vi "RMAD config.vi"() -> ()   [LabVIEW 2017]
panel:
  in  "Tab Control":T1(tab)
  out "Mote Status":T2(array[cluster]) {"mote state" items=["Lost"=0, "Negotiating"=1, "Operational"=4]}
  out "Link status":T3(array[cluster])
  in  "Send Reset":bool
  in  "SetAUX":bool
  in  "Node":u8=1
  in  "Get Status":bool
  in  "AUX min int":u16=15
  out "AUX data":T4(array[cluster]) {"Node configuration"."configuration" items=[""=100, "Repeater"=0, "Geofon"=1, "Sensor"=2, "Jernbane"=3, "Infralyd"=4]; "Node configuration"."radio config" items=[""=100, "Smartmesh IP"=0]; "batt(V)" format="%.3g"; "temp(c)" format="%.1g"; "?" format="%#.5g"}
  out "Is Logging":T5(array[cluster])
  in  "Adjustable Parameters":T6(array[cluster]) {"ACMP0 ch" items=["Geo 1"=0, "Geo 2"=3]; "ACMP1 ch" items=["Geo 3"=2, "Geo 4"=3]}
  in  "Get Adjustable Params":bool
  in  "Set adjust parameters":bool
  in  "Node":i32=1
  out "NGI Packets Dust":cluster{"MAc Adress":string, "data":string}[](array[cluster])
  out "dust manager mac adress":string
  out "mac adress":string[](array[string])
  out "radio IO":errorcluster
  in  "stop":bool
  out "iteration":i32
  out "gateway IP":T7={"serial_mux IP"="127.0.0.1", "serial_mux port"=9900}
  out "sec since last packet":dbl
  out "node names":string[](array[string])
  in  "initfile":string="rmad config svv.ini"
  in  "stress testing enabled":bool
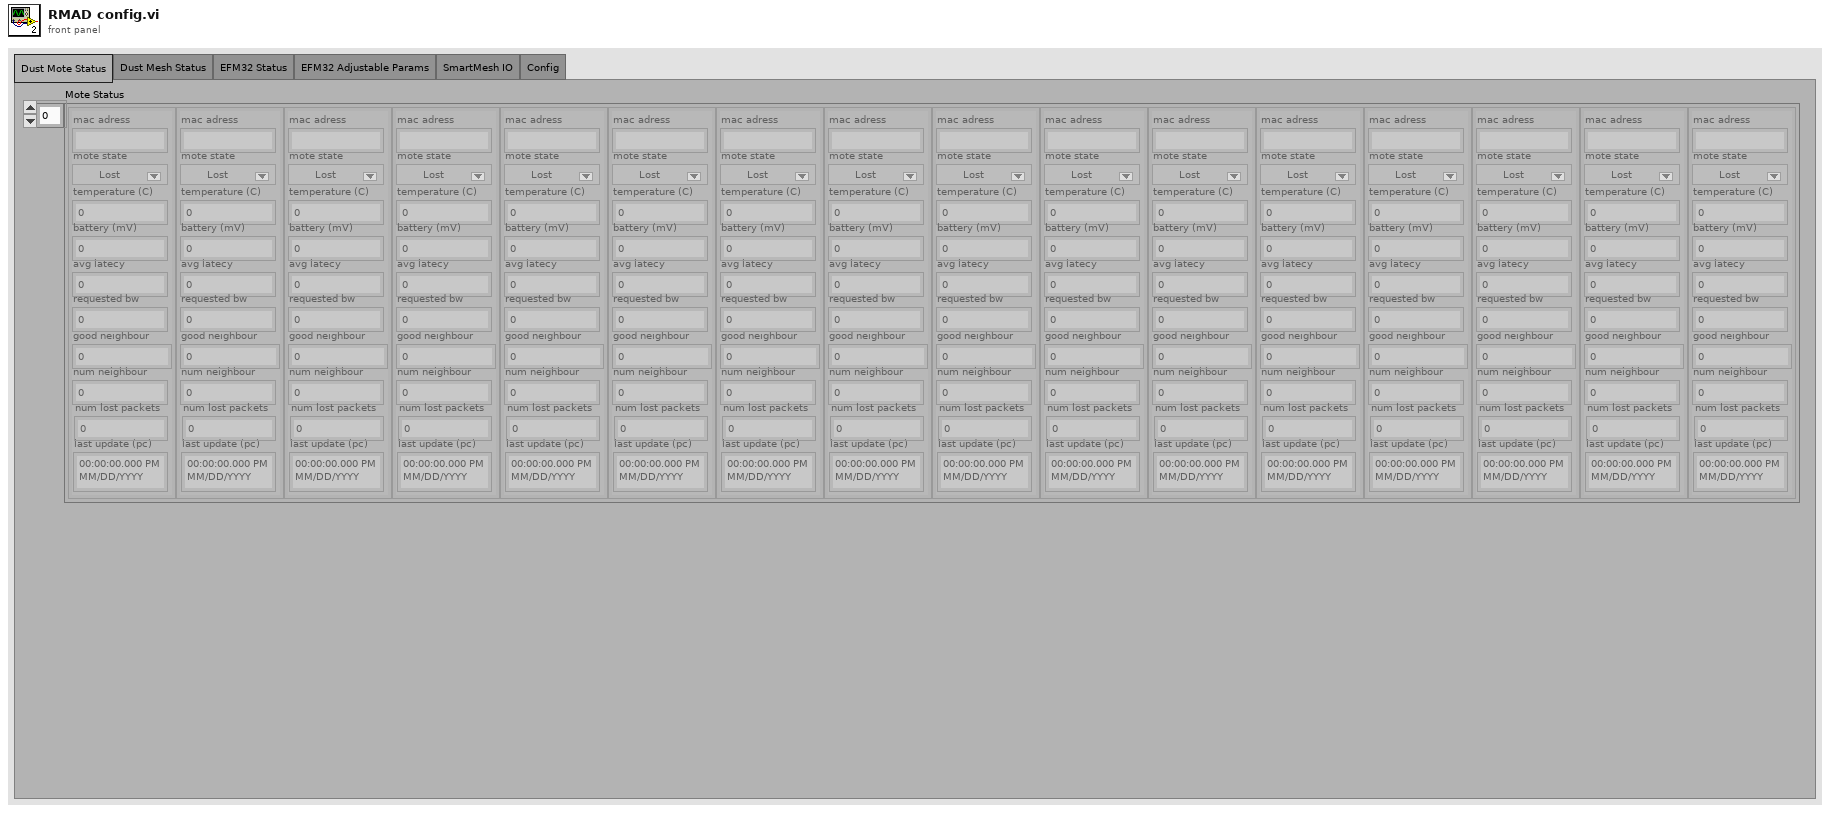
[diagram p1: front panel]
types:
  T1 = enum32{"Dust Mote Status", "Dust Mesh Status", "EFM32 Status", "EFM32 Adjustable Params", "SmartMesh IO", "Config"}
  T2 = cluster{"mac adress":string, "mote state":u8, "temperature (C)":i8, "battery (mV)":u16, "avg latecy":u32, "requested bw":u32, "good neighbour":u8, "num neighbour":u8, "num lost packets":u8, "last update (pc)":timestamp}[]
  T3 = cluster{"source mac adress":string, cluster{"destination":string, "rssi":i8, "TxPackets":u16}[], "last update":timestamp}[]
  T4 = cluster{"Node configuration":cluster{"configuration":u8, "sw ver":u8, "hw rev":u8, "radio config":u8}, "flaggs":bool[], "batt(V)":dbl, "temp(c)":dbl, "is singed int?":bool[], dbl[], "last update (pc)":timestamp}[]
  T5 = cluster{"Is logging":bool, "num avalanch":u16, "logging startet":timestamp}[]
  T6 = cluster{"Min samples":u32, "Samp after cont":u32, "Max samples":u32, "A1 std lim":sgl, "A2 std lim":sgl, "A3 std lim":sgl, "A4 std lim":sgl, "A1 cont lim":sgl, "A2 cont lim":sgl, "A3 cont lim":sgl, "A4 cont lim":sgl, "trigg level":u32, "sample delay":u32, "ACMP0 ch":u8, "ACMP1 ch":u8, "amp trigg":u16, "amp logging":u16}[]
  T7 = cluster{"serial_mux IP":string, "serial_mux port":u16}
  T8 = enum16{"big-endian, network order", "native, host order", "little-endian"}
  T9 = typedef "LVDateTimeRec.ctl" = cluster{"fractional second":dbl, "second":i32, "minute":i32, "hour":i32, "day of month":i32, "month":i32, "year":i32, "day of week":i32, "day of year":i32, "DST":i32}
  T10 = cluster{"Device Health Report":cluster{"MAC adress":string, "charge (mC)":u32, "queueOcc":u8, "temperature (C)":i8, "batteryVoltage (mV)":u16, "numTxOk":u16, "numTxFail":u16, "numRxOK":u16, "numRxFail":u16, "numMACdropped":u8, "numTxBad":u8, "badLinkFrameID":u8, "badLinkSlot":u32, "badLinkOffset":u8}, "mote staus event":cluster{"data":string, u8}, "getMoteInfo":cluster{"MAC adress":string, "state":u8, "numNbrs":u8, "numGoodNbrs":u8, "requestedBw":u32, "totalNeededBw":u32, "assignedBw":u32, "packetsRecived":u32, "packetsLost":u32, "avgLatecy":u32}, "GetPathInfo":cluster{"Path ID":u8, "Src MAC":string, "Dest MAC":string, "direction":u8, "numLinks":u8, "quality":u8, "rssiScrDest":i8, "rssiDestScr":i8}, "Neighbors Health Report":cluster{"MAC adress":string, "neighbourHRdata":cluster{"neighbourID":u16, "neighborFlag":u8, "rssi":i8, "numTxPackets":u16, "numTxFailures":u16, "numRxPackets":u16}[]}, "Discovered Nighbors Health Report":cluster{"MAC adress":string, "numJoinParents":u8, cluster{"neighborID":u16, "rssi":i8, "numRx":u8}[]}, "Mote Config":cluster{"mac adress":string, "MoteID":u16, "isAP":bool, "mote state":u8, "reserved":u8, "isRouting":bool}}
  T11 = cluster{"MAc Adress":string, "UTC Time":timestamp, "srcPort":u16, "dstPort":u16, "data":string}
  T12 = cluster{"Min samples":u32, "Samples after cont":u32, "Max samples":u32, "A1 std lim":sgl, "A2 std lim":sgl, "A3 std lim":sgl, "A4 std lim":sgl, "A1 cont lim":sgl, "A2 cont lim":sgl, "A3 cont lim":sgl, "A4 cont lim":sgl, "ACMP0 level":u32, "ACMP1 level":u32, "ACMP0 ch":u8, "ACMP1 ch":u8, "amp trigg":u16, "amp logging":u16}[]
  T13 = cluster{"Node configuration":cluster{"configuration":u8, "sw vertion":u8, "hw revition":u8, "radio config":u8}, "flaggs":bool[], "batteri (V)":dbl, "temperatur (c)":dbl, "is singed int?":bool[], dbl[], "last update (pc time)":timestamp}[]
  T14 = cluster{"source mac adress":string, cluster{"destination mac":string, "rssi":i8, "numTxPackets":u16}[], "last update":timestamp}[]
  T15 = cluster{"serial_mux IP":string, "rserial_mux port":u16}
  T16 = cluster{"dust master mac":string, "xbee master mac":string, "master name":string, "dust mac":string[], "xbee mac":string[], "node names":string[]}
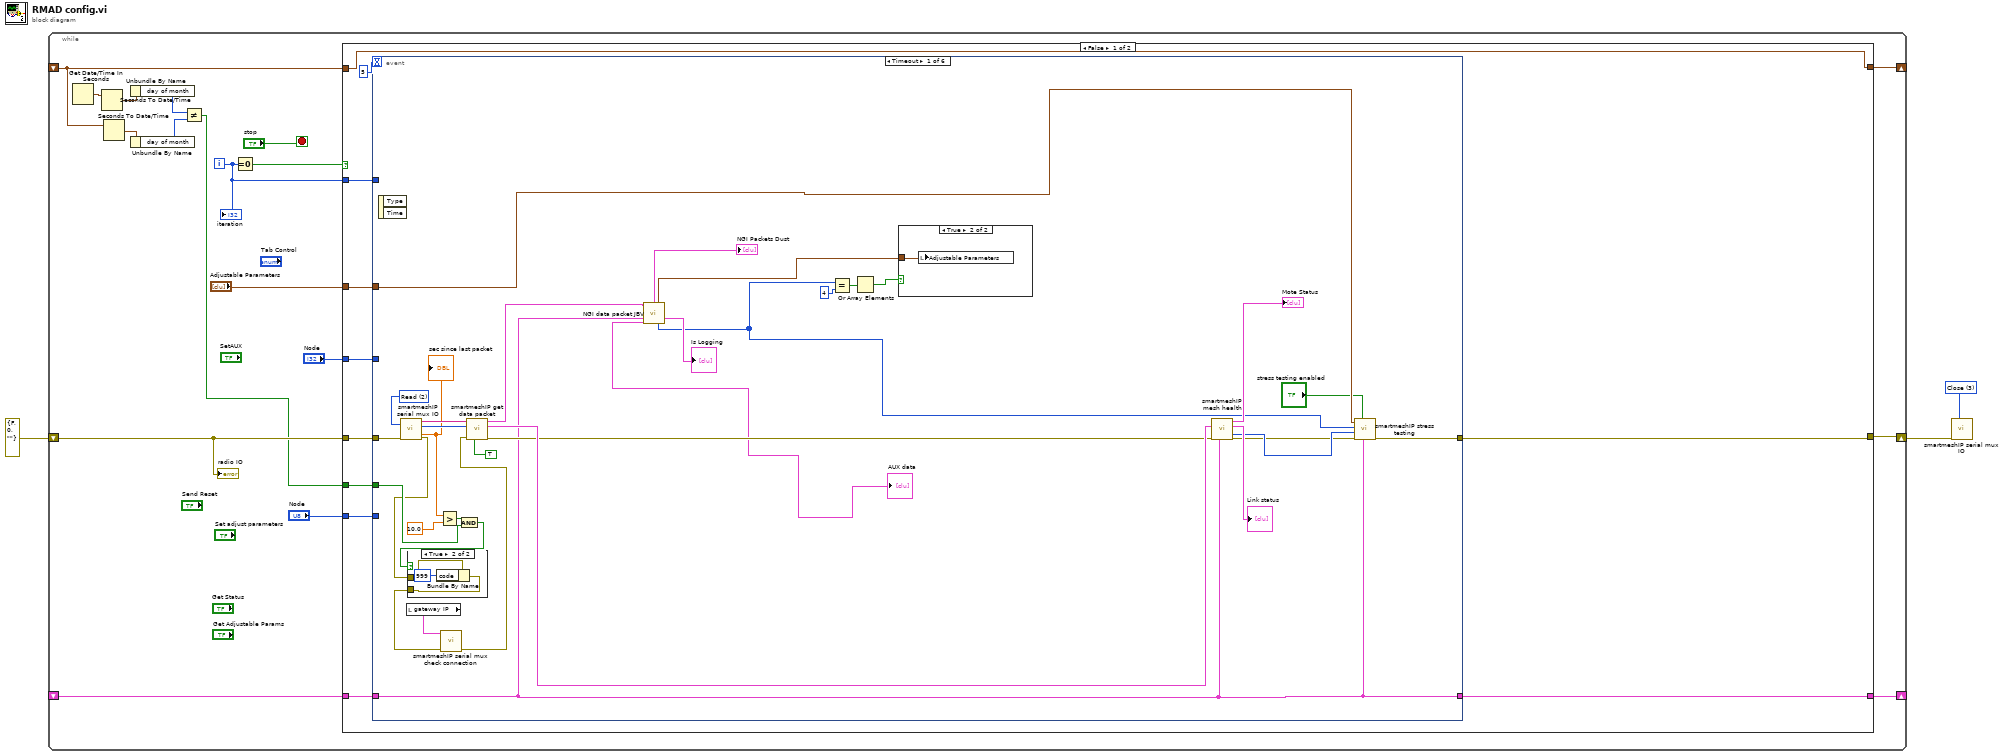
[diagram p0: block diagram]
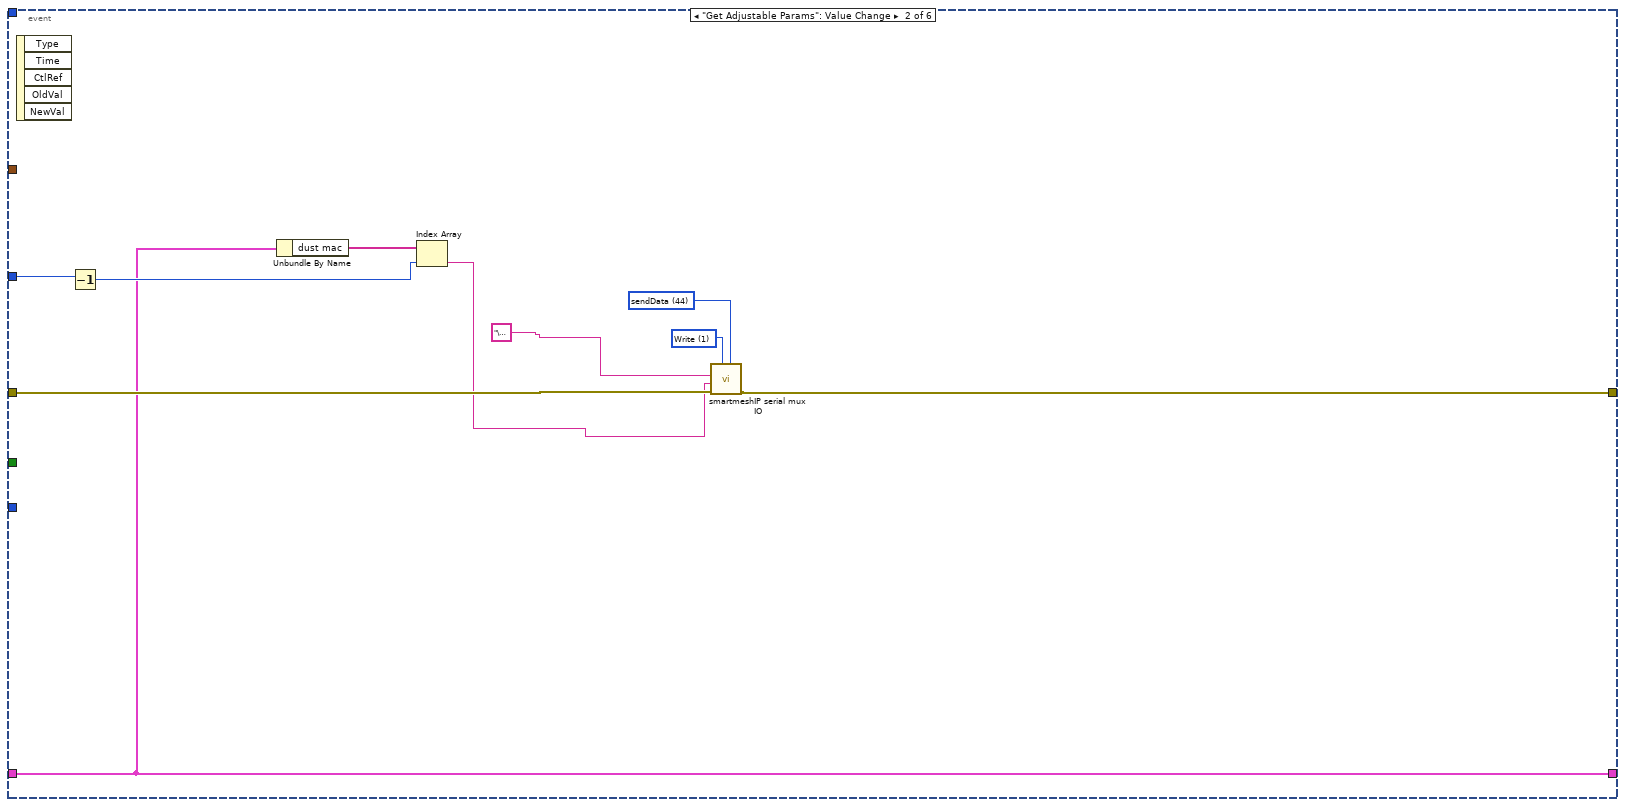
[diagram p4: hidden frame]
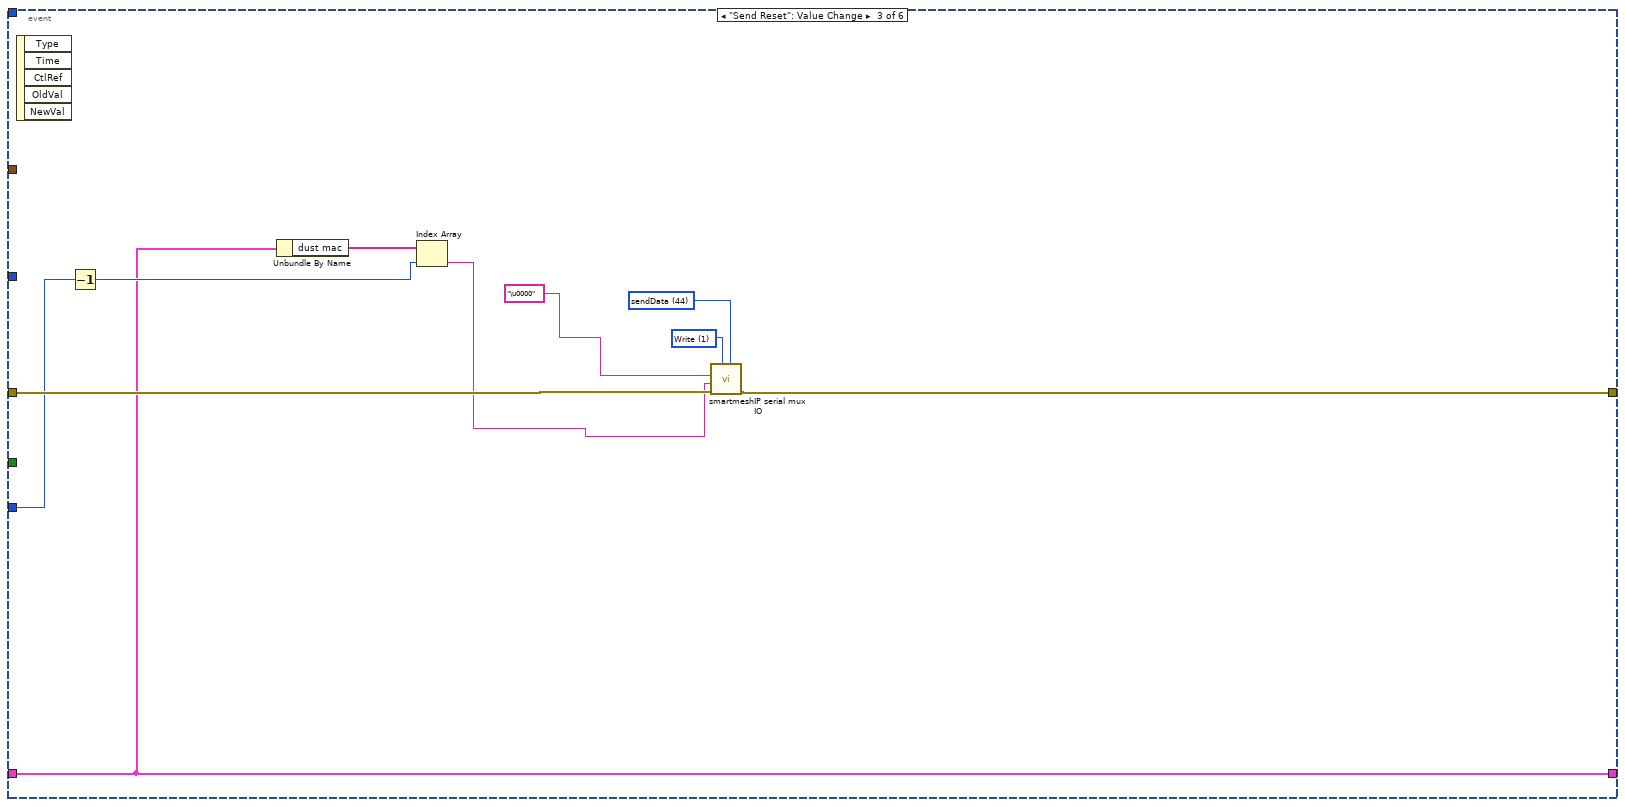
[diagram p5: hidden frame]
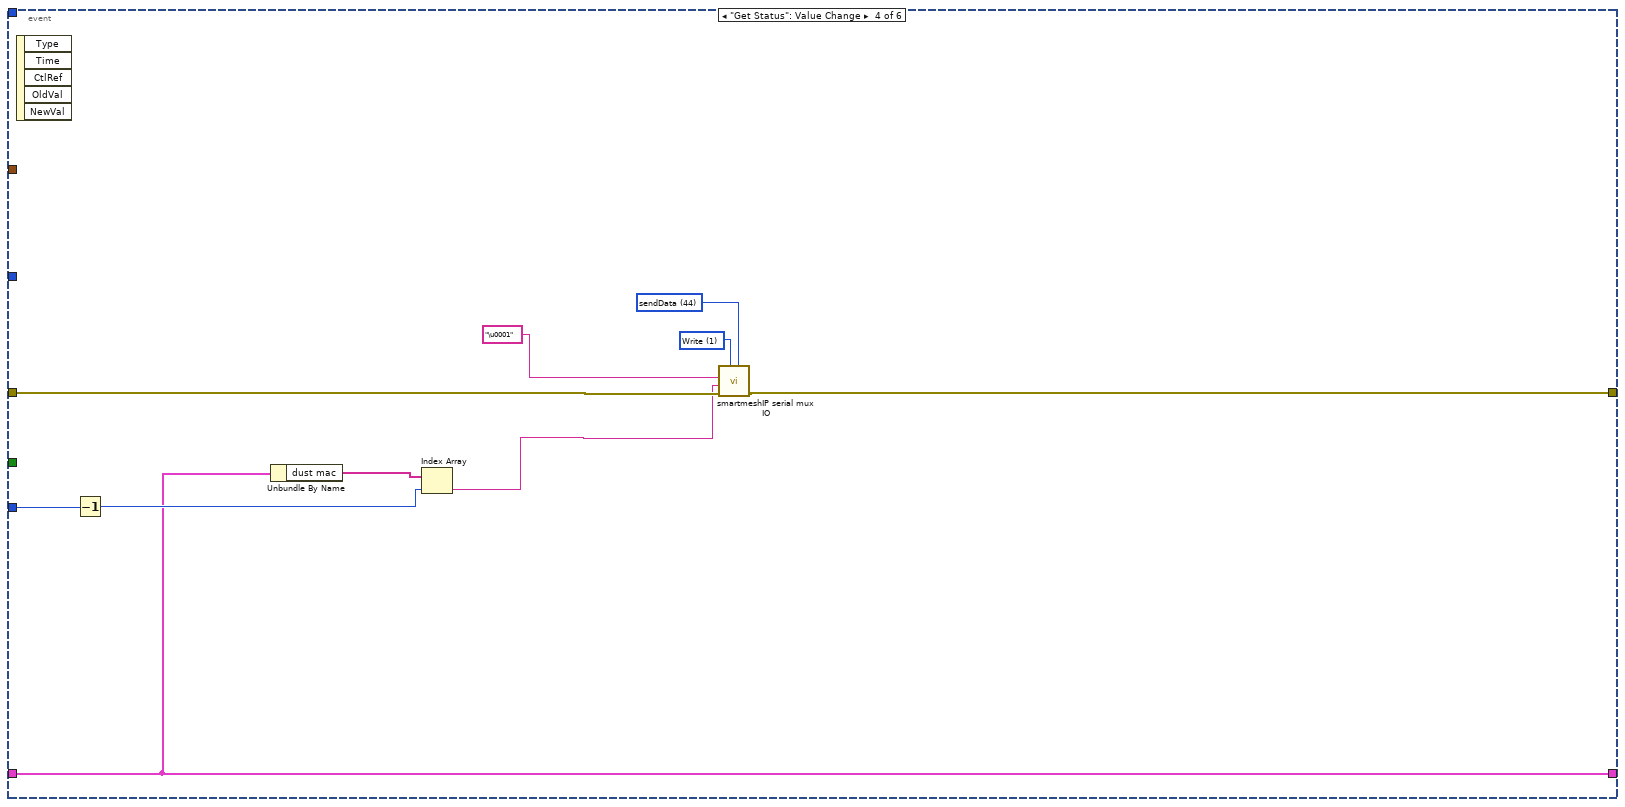
[diagram p6: hidden frame]
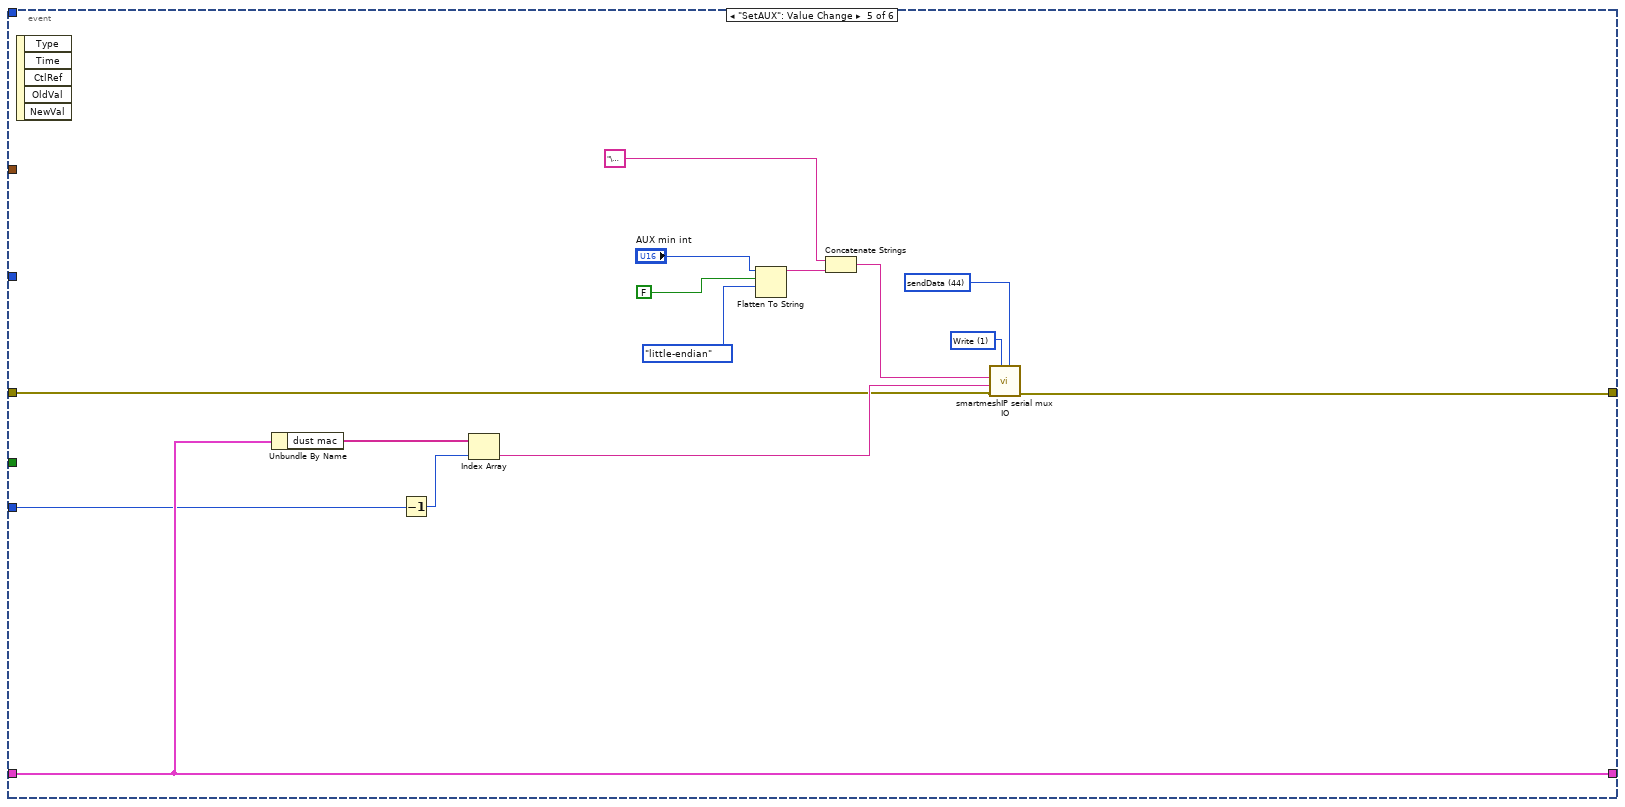
[diagram p7: hidden frame]
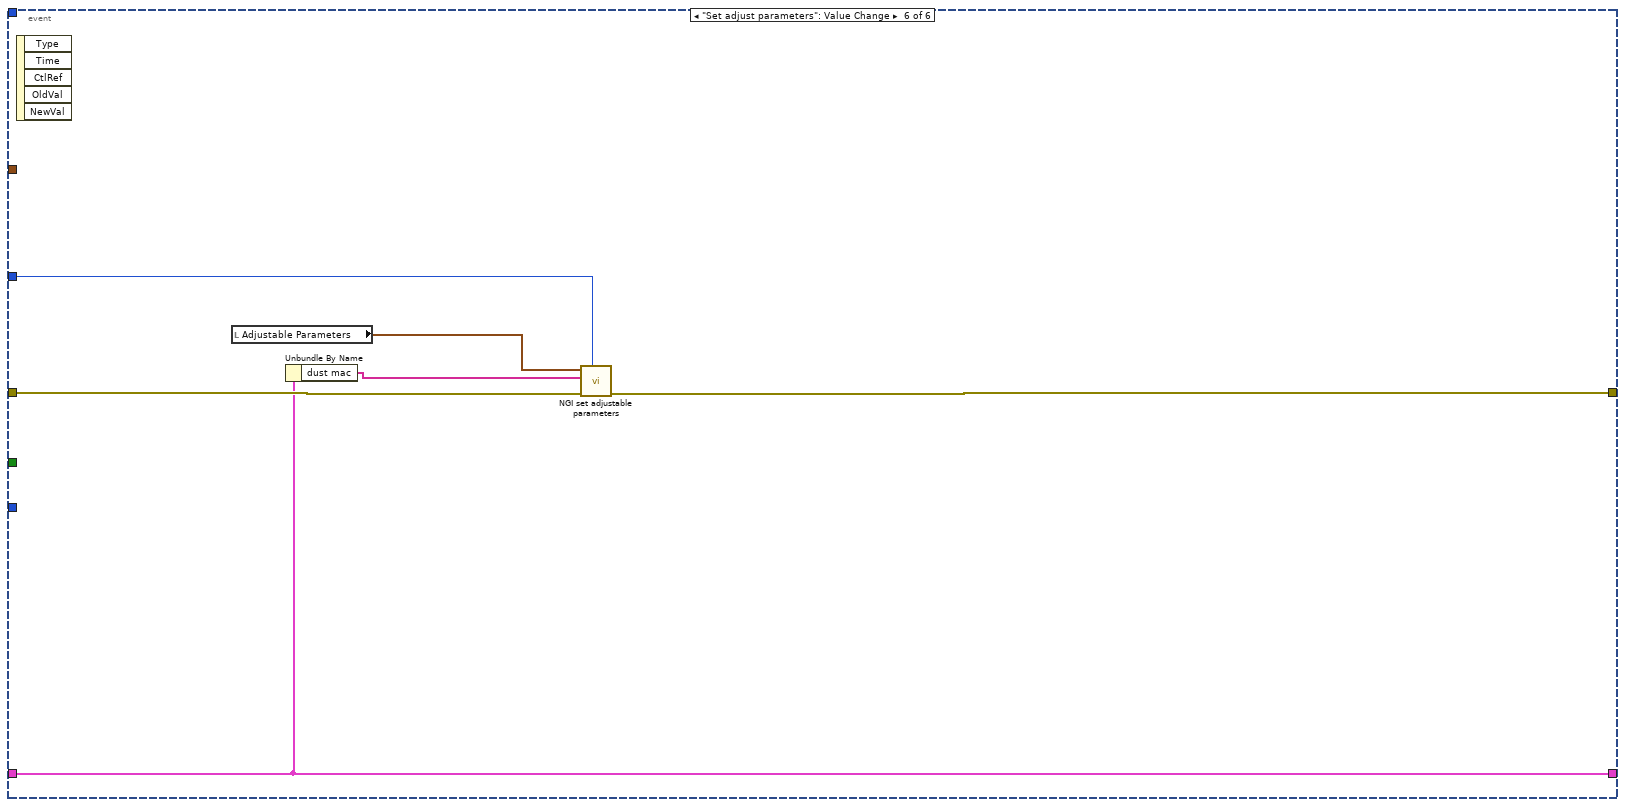
[diagram p8: hidden frame]
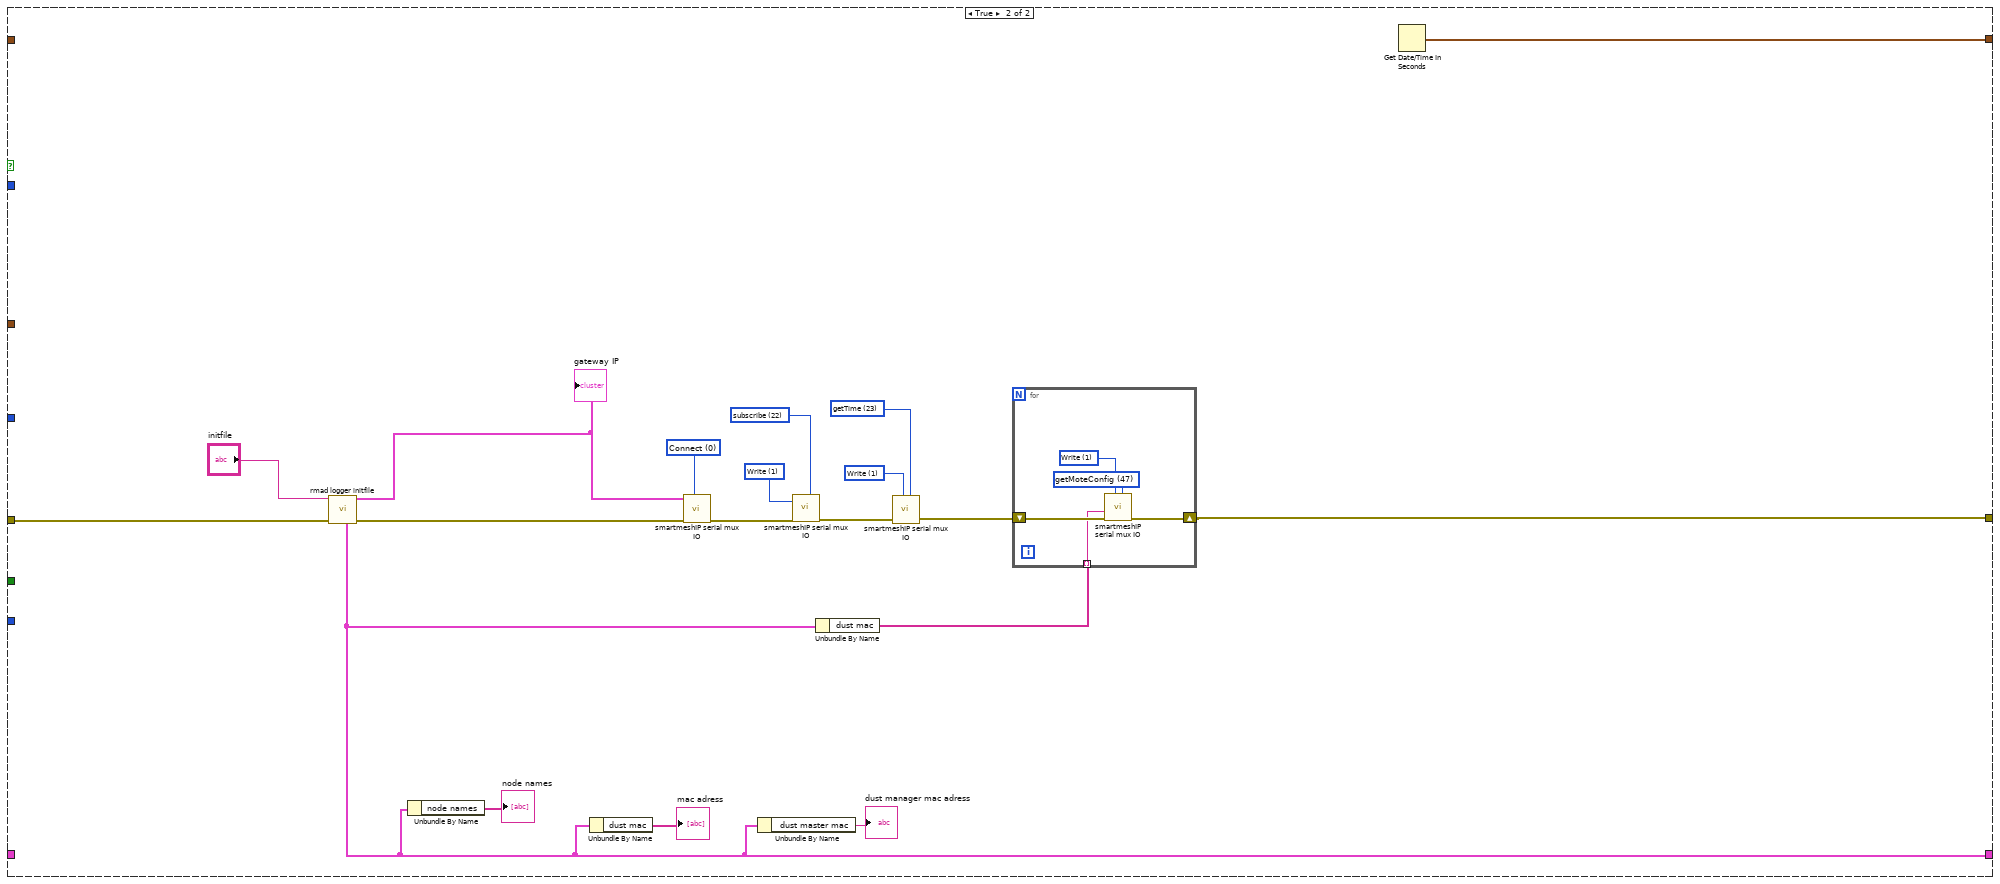
[diagram p9: hidden frame]
diagram:
  w3 = u16 3 items=["Connect", "Write", "Read", "Close"] ("State")
  n1 = while {
    shift-right: [w20] -> w2
    shift-left: errorcluster {"status"=FALSE, "code"=0, "source"=""} ("error out") -> [w14]
    shift-right: [w16] -> _
    shift-left: _ -> [w15]
    shift-right: [w11] -> _
    shift-left: _ -> [w4]
    i -> [w13]
    stop <- "stop" stop-if-true
    n2 = Get Date/Time In Seconds() -> (seconds since 1Jan1904=w6:timestamp)
    n3 = Seconds To Date/Time(time stamp (now)=w6) -> (date time rec=w10:T9)  [unwired: 1 in]
    n4 = Seconds To Date/Time(time stamp (now)=w4) -> (date time rec=w9:T9)  [unwired: 1 in]
    n5 = Unbundle By Name(w10) -> ("day of month"=w8:i32)
    n6 = Unbundle By Name(w9) -> ("day of month"=w7:i32)
    n7 = Not Equal?(x=w8, y=w7) -> (x != y?=w5:bool)
    n8 = Equal To 0?(x=w13) -> (x = 0?=w21:bool)
    n9 = case shown="False" w21 {
      tunnel: [w23 w124] -> w20
      tunnel: w14 -> [w32 w123]
      tunnel: w13 -> [w30 _]
      tunnel: "Node" -> [w29 _]
      tunnel: "Node" -> [w28 _]
      tunnel: [w25 w126] -> w16
      tunnel: w15 -> [w27 _]
      tunnel: "Adjustable Parameters" -> [w26 _]
      tunnel: [w22 w128] -> w11
      tunnel: w4 -> [w22 _]
      tunnel: w5 -> [w24 _]
      frame False {
        n10 = event shown="[0] Timeout" {
          selector: _ -> [_ _ _ _ _ _]
          dyn-events: _ -> [_ _ _ _ _ _]
          timeout: 5 -> [_ _ _ _ _ _]
          tunnel: w32 -> [w65 w76 w87 w96 w110 w121]
          tunnel: [w52 w75 w86 w93 w106 w120] -> w23
          tunnel: w30 -> [_ _ _ _ _ _]
          tunnel: w29 -> [_ _ w81 w100 w103 _]
          tunnel: w28 -> [_ w79 _ _ _ w118]
          tunnel: w27 -> [w38 w72 w84 w92 w108 w116]
          tunnel: [w38 w72 w84 w92 w108 w116] -> w25
          tunnel: w26 -> [w50 _ _ _ _ _]
          tunnel: w24 -> [w46 _ _ _ _ _]
          event Timeout {
            w64 = u16 2 items=["Connect", "Write", "Read", "Close"] ("State")
            n11 = event-data() -> ()  [unwired: 1 in, 2 out]
            n12 = call "smartmeshIP serial mux IO.vi"("State"=w64, "error in"=w65) -> ("error out"=w44:errorcluster, "rx_commandType"=w59:u8, "rx_data"=w60:string, "sec since last packet"=w49:dbl)  [unwired: 4 in, 2 out]
            "sec since last packet" <- w49
            n13 = local read "gateway IP"() -> (w54:T7)
            n14 = Greater?(x=w49, y=10.0) -> (0:w47:bool)
            n15 = And(x=w47, y=w46) -> (x .and. y?=w45:bool)
            n16 = case shown="True" w45 {
              tunnel: w44 -> [w66 w69]
              tunnel: [w66 w68] -> w43
              frame False {
              }
              frame True {
                n17 = Bundle By Name(cluster=w69, "code"=999) -> (w68:errorcluster)
              }
            }
            n18 = call "smartmeshIP serial mux check connection.vi"("error in"=w43, "serial mux adress"=w54) -> ("error out"=w53:errorcluster)  [unwired: 8 in, 1 out]
            n19 = call "smartmeshIP get data packet.vi"("use correction"=TRUE ("use time correction"), "error in"=w53, "commandType"=w59, "data"=w60) -> ("error out"=w42:errorcluster, "mote and link status"=w58:T10, "Data Notifications"=w39:T11)  [unwired: 5 in]
            n20 = call "NGI data packet JBV.vi"("Dust Data Notifications"=w39, "mac adresses"=w38) -> ("NGI  packets dust"=→"NGI Packets Dust":cluster{"MAc Adress":string, "data":string}[], "Adjustable Parameters"=w34:T12, "Is Logging"=→"Is Logging":T5, "AUX data"=→"AUX data":T13, "last packet type"=w35:u8[])  [unwired: 4 in, 5 out]
            n21 = Equal?(x=w35, y=u8 4) -> (x = y?=w62:bool[])
            n22 = Or Array Elements(Boolean array=w62) -> (logical OR=w61:bool)
            n23 = case shown="True" w61 {
              tunnel: w34 -> [_ w70]
              frame False {
              }
              frame True {
                n24 = local write "Adjustable Parameters"(w70) -> ()
              }
            }
            n25 = call "smartmeshIP mesh health.vi"("mote and link status"=w58, "error in"=w42, "mac adresses"=w38) -> ("Mote Status"=→"Mote Status":T2, "Primary link status"=→"Link status":T14, "last packet type dust"=w51:i32[], "error out"=w41:errorcluster)  [unwired: 7 in, 2 out]
            n26 = call "smartmeshIP stress testing.vi"("mac adresses"=w38, "stress testing enabled"="stress testing enabled", "error in"=w41, "last packet type dust"=w51, "last packet type ngi"=w35, "Adjustable Parameters"=w50) -> ("error out"=w52:errorcluster)  [unwired: 5 in]
          }
          event "Get Adjustable Params": Value Change {
            w78 = u8 44 items=["subscribe"=22, "startNetwork"=45, "setUser"=58, "setTime"=54, "setNetworkConfig"=26, "setLicense"=56, "setIPConfig"=68, "setDownstreamFrameMode"=51, "setCommonJoinKey"=66, "setAdvertising"=50, "setACLEntry"=39, "sendIP"=59, "sendData"=44, "restorFactoryDefaults"=61, "reset"=21, "radiotestTx"=35, "radiotestRx"=37, "pingMote"=42, "getTime"=23, "getSystemInfo"=46, "radiotestStatistics"=38, "getPathInfo"=48, "getNextPath"=49, "getNextACLEntry"=40, "getNetworkInfo"=64, "getNetworkConfig"=63, "getMoteLinks"=70, "getMoteInfo"=62, "getMoteConfigByld"=65, "getMoteConfig"=47, "getManagerStatistics"=53, "getLog"=43, "getLicense"=55, "getIPConfig"=67, "exchangeNetworkID"=34, "exchangeMoteJoinKey"=33, "deleteMote"=69, "deleteACLEntry"=41, "clearStatistics"=31] ("commandType_write")
            w77 = u16 1 items=["Connect", "Write", "Read", "Close"] ("State")
            n27 = event-data() -> ()  [unwired: 1 in, 5 out]
            n28 = Decrement(x=w79) -> (x-1=w80:i32)
            n29 = Unbundle By Name(w72) -> ("dust mac"=w71:string[])
            n30 = Index Array(array=w71, index=w80) -> (element=w73:string)
            n31 = call "smartmeshIP serial mux IO.vi"("tx_commandType"=w78, "State"=w77, "error in"=w76, "MAC source"=w73, "tx_data"="\u0005") -> ("error out"=w75:errorcluster)  [unwired: 1 in, 5 out]
          }
          event "Send Reset": Value Change {
            w89 = u8 44 items=["subscribe"=22, "startNetwork"=45, "setUser"=58, "setTime"=54, "setNetworkConfig"=26, "setLicense"=56, "setIPConfig"=68, "setDownstreamFrameMode"=51, "setCommonJoinKey"=66, "setAdvertising"=50, "setACLEntry"=39, "sendIP"=59, "sendData"=44, "restorFactoryDefaults"=61, "reset"=21, "radiotestTx"=35, "radiotestRx"=37, "pingMote"=42, "getTime"=23, "getSystemInfo"=46, "radiotestStatistics"=38, "getPathInfo"=48, "getNextPath"=49, "getNextACLEntry"=40, "getNetworkInfo"=64, "getNetworkConfig"=63, "getMoteLinks"=70, "getMoteInfo"=62, "getMoteConfigByld"=65, "getMoteConfig"=47, "getManagerStatistics"=53, "getLog"=43, "getLicense"=55, "getIPConfig"=67, "exchangeNetworkID"=34, "exchangeMoteJoinKey"=33, "deleteMote"=69, "deleteACLEntry"=41, "clearStatistics"=31] ("commandType_write")
            w88 = u16 1 items=["Connect", "Write", "Read", "Close"] ("State")
            n32 = event-data() -> ()  [unwired: 1 in, 5 out]
            n33 = Decrement(x=w81) -> (x-1=w90:u8)
            n34 = Unbundle By Name(w84) -> ("dust mac"=w83:string[])
            n35 = Index Array(array=w83, index=w90) -> (element=w85:string)
            n36 = call "smartmeshIP serial mux IO.vi"("tx_commandType"=w89, "State"=w88, "error in"=w87, "MAC source"=w85, "tx_data"="\u0000") -> ("error out"=w86:errorcluster)  [unwired: 1 in, 5 out]
          }
          event "Get Status": Value Change {
            w98 = u8 44 items=["subscribe"=22, "startNetwork"=45, "setUser"=58, "setTime"=54, "setNetworkConfig"=26, "setLicense"=56, "setIPConfig"=68, "setDownstreamFrameMode"=51, "setCommonJoinKey"=66, "setAdvertising"=50, "setACLEntry"=39, "sendIP"=59, "sendData"=44, "restorFactoryDefaults"=61, "reset"=21, "radiotestTx"=35, "radiotestRx"=37, "pingMote"=42, "getTime"=23, "getSystemInfo"=46, "radiotestStatistics"=38, "getPathInfo"=48, "getNextPath"=49, "getNextACLEntry"=40, "getNetworkInfo"=64, "getNetworkConfig"=63, "getMoteLinks"=70, "getMoteInfo"=62, "getMoteConfigByld"=65, "getMoteConfig"=47, "getManagerStatistics"=53, "getLog"=43, "getLicense"=55, "getIPConfig"=67, "exchangeNetworkID"=34, "exchangeMoteJoinKey"=33, "deleteMote"=69, "deleteACLEntry"=41, "clearStatistics"=31] ("commandType_write")
            w97 = u16 1 items=["Connect", "Write", "Read", "Close"] ("State")
            n37 = event-data() -> ()  [unwired: 1 in, 5 out]
            n38 = Decrement(x=w100) -> (x-1=w99:u8)
            n39 = Unbundle By Name(w92) -> ("dust mac"=w91:string[])
            n40 = Index Array(array=w91, index=w99) -> (element=w94:string)
            n41 = call "smartmeshIP serial mux IO.vi"("tx_commandType"=w98, "State"=w97, "error in"=w96, "MAC source"=w94, "tx_data"="\u0001") -> ("error out"=w93:errorcluster)  [unwired: 1 in, 5 out]
          }
          event "SetAUX": Value Change {
            w113 = u8 44 items=["subscribe"=22, "startNetwork"=45, "setUser"=58, "setTime"=54, "setNetworkConfig"=26, "setLicense"=56, "setIPConfig"=68, "setDownstreamFrameMode"=51, "setCommonJoinKey"=66, "setAdvertising"=50, "setACLEntry"=39, "sendIP"=59, "sendData"=44, "restorFactoryDefaults"=61, "reset"=21, "radiotestTx"=35, "radiotestRx"=37, "pingMote"=42, "getTime"=23, "getSystemInfo"=46, "radiotestStatistics"=38, "getPathInfo"=48, "getNextPath"=49, "getNextACLEntry"=40, "getNetworkInfo"=64, "getNetworkConfig"=63, "getMoteLinks"=70, "getMoteInfo"=62, "getMoteConfigByld"=65, "getMoteConfig"=47, "getManagerStatistics"=53, "getLog"=43, "getLicense"=55, "getIPConfig"=67, "exchangeNetworkID"=34, "exchangeMoteJoinKey"=33, "deleteMote"=69, "deleteACLEntry"=41, "clearStatistics"=31] ("commandType_write")
            w112 = u16 1 items=["Connect", "Write", "Read", "Close"] ("State")
            n42 = event-data() -> ()  [unwired: 1 in, 5 out]
            n43 = Unbundle By Name(w108) -> ("dust mac"=w107:string[])
            n44 = Decrement(x=w103) -> (x-1=w109:u8)
            n45 = Index Array(array=w107, index=w109) -> (element=w111:string)
            n46 = Flatten To String(anything="AUX min int", prepend array or string size? (T)=FALSE, byte order (0:big-endian, network order)=T8."little-endian") -> (data string=w104:string)  [unwired: 1 in, 2 out]
            n47 = Concatenate Strings("\u000b", w104) -> (w101:string)
            n48 = call "smartmeshIP serial mux IO.vi"("tx_commandType"=w113, "State"=w112, "error in"=w110, "MAC source"=w111, "tx_data"=w101) -> ("error out"=w106:errorcluster)  [unwired: 1 in, 5 out]
          }
          event "Set adjust parameters": Value Change {
            n49 = event-data() -> ()  [unwired: 1 in, 5 out]
            n50 = local read "Adjustable Parameters"() -> (w119:T6)
            n51 = Unbundle By Name(w116) -> ("dust mac"=w117:string[])
            n52 = call "NGI set adjustable parameters.vi"("node nummer"=w118, "error in"=w121, "dust mac adress"=w117, "Adjustable Parameters"=w119) -> ("error out"=w120:errorcluster)  [unwired: 7 in]
          }
        }
      }
      frame True {
        w134 = u8 23 items=["subscribe"=22, "startNetwork"=45, "setUser"=58, "setTime"=54, "setNetworkConfig"=26, "setLicense"=56, "setIPConfig"=68, "setDownstreamFrameMode"=51, "setCommonJoinKey"=66, "setAdvertising"=50, "setACLEntry"=39, "sendIP"=59, "sendData"=44, "restorFactoryDefaults"=61, "reset"=21, "radiotestTx"=35, "radiotestRx"=37, "pingMote"=42, "getTime"=23, "getSystemInfo"=46, "radiotestStatistics"=38, "getPathInfo"=48, "getNextPath"=49, "getNextACLEntry"=40, "getNetworkInfo"=64, "getNetworkConfig"=63, "getMoteLinks"=70, "getMoteInfo"=62, "getMoteConfigByld"=65, "getMoteConfig"=47, "getManagerStatistics"=53, "getLog"=43, "getLicense"=55, "getIPConfig"=67, "exchangeNetworkID"=34, "exchangeMoteJoinKey"=33, "deleteMote"=69, "deleteACLEntry"=41, "clearStatistics"=31] ("commandType_write")
        w135 = u16 1 items=["Connect", "Write", "Read", "Close"] ("State")
        w137 = u8 22 items=["subscribe"=22, "startNetwork"=45, "setUser"=58, "setTime"=54, "setNetworkConfig"=26, "setLicense"=56, "setIPConfig"=68, "setDownstreamFrameMode"=51, "setCommonJoinKey"=66, "setAdvertising"=50, "setACLEntry"=39, "sendIP"=59, "sendData"=44, "restorFactoryDefaults"=61, "reset"=21, "radiotestTx"=35, "radiotestRx"=37, "pingMote"=42, "getTime"=23, "getSystemInfo"=46, "radiotestStatistics"=38, "getPathInfo"=48, "getNextPath"=49, "getNextACLEntry"=40, "getNetworkInfo"=64, "getNetworkConfig"=63, "getMoteLinks"=70, "getMoteInfo"=62, "getMoteConfigByld"=65, "getMoteConfig"=47, "getManagerStatistics"=53, "getLog"=43, "getLicense"=55, "getIPConfig"=67, "exchangeNetworkID"=34, "exchangeMoteJoinKey"=33, "deleteMote"=69, "deleteACLEntry"=41, "clearStatistics"=31] ("commandType_write")
        w138 = u16 1 items=["Connect", "Write", "Read", "Close"] ("State")
        w140 = u16 0 items=["Connect", "Write", "Read", "Close"] ("State")
        n53 = call "rmad logger initfile.vi"("initfile"="initfile", "error in (no error)"=w123) -> ("serial mux"=w125:T15, "mac adresses"=w126:T16, "error out"=w129:errorcluster)  [unwired: 1 in, 10 out]
        "gateway IP" <- w125
        n54 = Unbundle By Name(w126) -> ("node names"=→"node names":string[])
        n55 = Unbundle By Name(w126) -> ("dust mac"=→"mac adress":string[])
        n56 = call "smartmeshIP serial mux IO.vi"("State"=w140, "error in"=w129, "serial mux adress"=w125) -> ("error out"=w139:errorcluster)  [unwired: 3 in, 5 out]
        n57 = Unbundle By Name(w126) -> ("dust master mac"=→"dust manager mac adress":string)
        n58 = call "smartmeshIP serial mux IO.vi"("tx_commandType"=w137, "State"=w138, "error in"=w139) -> ("error out"=w136:errorcluster)  [unwired: 3 in, 5 out]
        n59 = Unbundle By Name(w126) -> ("dust mac"=w132:string[])
        n60 = call "smartmeshIP serial mux IO.vi"("tx_commandType"=w134, "State"=w135, "error in"=w136) -> ("error out"=w133:errorcluster)  [unwired: 3 in, 5 out]
        n61 = for {
          shift-right: [w142] -> w124
          shift-left: w133 -> [w143]
          tunnel: w132 -> [w141] mode=indexing
          w145 = u16 1 items=["Connect", "Write", "Read", "Close"] ("State")
          w144 = u8 47 items=["subscribe"=22, "startNetwork"=45, "setUser"=58, "setTime"=54, "setNetworkConfig"=26, "setLicense"=56, "setIPConfig"=68, "setDownstreamFrameMode"=51, "setCommonJoinKey"=66, "setAdvertising"=50, "setACLEntry"=39, "sendIP"=59, "sendData"=44, "restorFactoryDefaults"=61, "reset"=21, "radiotestTx"=35, "radiotestRx"=37, "pingMote"=42, "getTime"=23, "getSystemInfo"=46, "radiotestStatistics"=38, "getPathInfo"=48, "getNextPath"=49, "getNextACLEntry"=40, "getNetworkInfo"=64, "getNetworkConfig"=63, "getMoteLinks"=70, "getMoteInfo"=62, "getMoteConfigByld"=65, "getMoteConfig"=47, "getManagerStatistics"=53, "getLog"=43, "getLicense"=55, "getIPConfig"=67, "exchangeNetworkID"=34, "exchangeMoteJoinKey"=33, "deleteMote"=69, "deleteACLEntry"=41, "clearStatistics"=31] ("commandType_write")
          n62 = call "smartmeshIP serial mux IO.vi"("tx_commandType"=w144, "State"=w145, "error in"=w143, "MAC source"=w141) -> ("error out"=w142:errorcluster)  [unwired: 2 in, 5 out]
        }
        n63 = Get Date/Time In Seconds() -> (seconds since 1Jan1904=w128:timestamp)
      }
    }
    "radio IO" <- w14
    "iteration" <- w13
  }
  n64 = call "smartmeshIP serial mux IO.vi"("State"=w3, "error in"=w2) -> ()  [unwired: 4 in, 6 out]
